vi "Open Project if Not in Memory.vi"(8 "error in (no error)":errorcluster, 11 "Path":path) -> (0 "error out":errorcluster, 3 "Project Ref":refnum<vi>, 5 "Opened?":bool)   [LabVIEW 2020, in "VI Properties Editor.lvlib"]
doc: "Opens the project specified by <B>Path</B> only if it was not already in memory."
uses:
  VI Properties Editor.lvlib
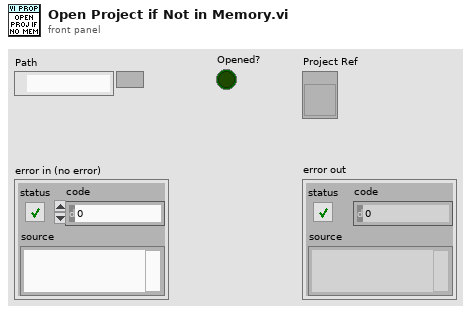
[diagram p1: front panel]
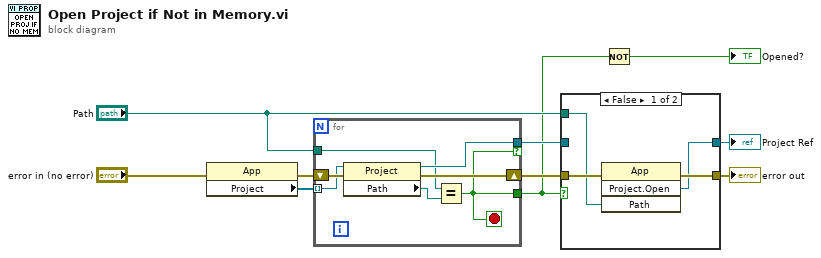
[diagram p0: block diagram]
diagram:
  n1 = property on="Property Node" class="App"(error in="error in (no error)") -> (error out=w10:errorcluster, "Project"=w8:refnum<vi>[])  [unwired: 1 in, 1 out]
  n2 = for {
    tunnel: w8 -> [w15] mode=indexing
    tunnel: "Path" -> [w11]
    tunnel: [w13] -> w7 if=w12
    tunnel: [w12] -> w3
    shift-right: [w16] -> w9
    shift-left: w10 -> [w17]
    stop <- w12 stop-if-true
    n3 = property on="Property Node" class="Project"(reference=w15, error in=w17) -> (reference out=w13:refnum<vi>, error out=w16:errorcluster, "Path"=w14:path)
    n4 = Equal?(x=w11, y=w14) -> (x = y?=w12:bool)
  }
  n5 = case shown="False" w3 {
    tunnel: [w21 w23] -> w5
    tunnel: [w19 w22] -> w4
    tunnel: w7 -> [_ w22]
    tunnel: "Path" -> [w18 _]
    tunnel: w9 -> [w20 w23]
    frame False {
      n6 = invoke on="Invoke Node" class="App" method="Project.Open"(error in=w20, "Path"=w18) -> (error out=w21:errorcluster, "Project:Open"=w19:refnum<vi>)  [unwired: 2 in, 2 out]
    }
    frame True {
    }
  }
  "error out" <- w5
  "Project Ref" <- w4
  n7 = Not(x=w3) -> (.not. x?=→"Opened?":bool)
